vi "Logger-Get Log Text.vi"(11 "error in (no error)":errorcluster) -> (6 "name":string, 8 "text":string, 15 "error out":errorcluster)   [LabVIEW 2020]
uses:
  Typedefs/Logger-Queue Data.ctl
  Typedefs/Logger-Action.ctl
  Typedefs/Logger-Level.ctl
  Controls/Utilities-Wait.vi/89bc9713-8f2c-40bd-a11f-1c800a437687.vi
  <vilib>/Utility/High Resolution Polling Wait.vi
  Typedefs/Logger-Globals.vi
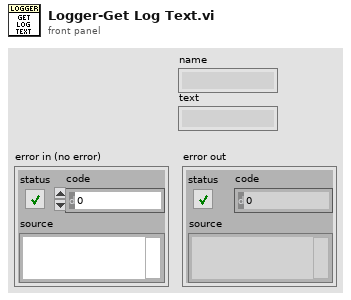
[diagram p1: front panel]
types:
  T1 = typedef "Logger-Action.ctl" = enum16{"None", "Init", "Add", "Show", "Quit"}
  T2 = typedef "Logger-Queue Data.ctl" = cluster{"Action":T1, "Level":T3, "Time":dbl, "Message":string}
  T3 = typedef "Logger-Level.ctl" = enum16{"Debug", "TCP", "Info", "Warning", "Error", "Critical"}
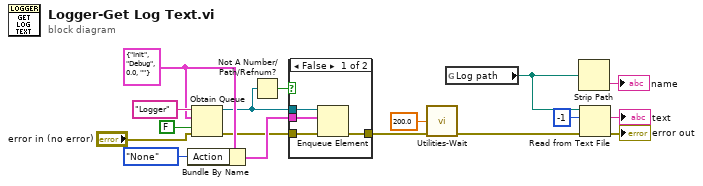
[diagram p0: block diagram]
diagram:
  w13 = T2 {"Action"=enum."Init", "Level"=enum."Debug", "Time"=0.0, "Message"=""} ("Trace Data")
  n1 = Bundle By Name(cluster=w13, "Action"=Logger-Action."None") -> (w11:T2)
  n2 = Obtain Queue(name (unnamed)="Logger", element data type=w13, create if not found? (T)=FALSE, error in (no error)="error in (no error)") -> (queue out=w9:refnum<queue>, error out=w10:errorcluster)  [unwired: 1 in, 1 out]
  n3 = Not A Number/Path/Refnum?(number/path/refnum=w9) -> (NaN/Path/Refnum?=w8:bool)
  n4 = case shown="False" w8 {
    tunnel: w11 -> [w21 _]
    tunnel: w10 -> [w20 _]
    tunnel: w9 -> [w19 _]
    tunnel: [w18 _] -> w6
    frame False {
      n5 = Enqueue Element(queue=w19, element=w21, error in (no error)=w20) -> (error out=w18:errorcluster)  [unwired: 1 in, 2 out]
    }
    frame True {
    }
  }
  n6 = call "Utilities-Wait.vi"("milliseconds to wait"=200.0, "error in (no error)"=w6) -> ("error out"=w4:errorcluster)  [unwired: 13 in]
  n7 = global read "Logger-Globals.vi" "Log path"() -> (w2:path)
  n8 = Strip Path(path=w2) -> (name=→"name":string)  [unwired: 1 out]
  n9 = Read from Text File(file (use dialog)=w2, count=-1, error in=w4) -> (text=→"text":string, error out=→"error out":errorcluster)  [unwired: 1 in, 2 out]
